vi "Pre Parse Rules.vi"(8 "Error in":errorcluster, 10 "Rules String":string) -> (0 "Error out":errorcluster, 2 "Processed Rules":T1[](array[typedef]))   [LabVIEW 2019, in "LSS.lvlib"]
doc: "Takes the Rules String and splits it into a list of properties that can be used by the property control engine.\n\n<b>Inputs:</b>\n<b>Rules String</b> - Properly formatted string that will control the front panel by applying LSS.\n<b>Error In</b> - Standard Error In terminal.\n\n<b>Outputs:</b>\n<b>Processed Rules</b> - Cluster of criteria and effects that are defined by the Rules String.\n<b>Error Out</b> - Standard Error out terminal."
uses:
  LSS.lvlib
  Controls/Rule.ctl
  Controls/Criteria.ctl
  Controls/Comparison Types.ctl
  Controls/Effects.ctl
panel:
  out "Troubleshooting output only":string[][](array[string])
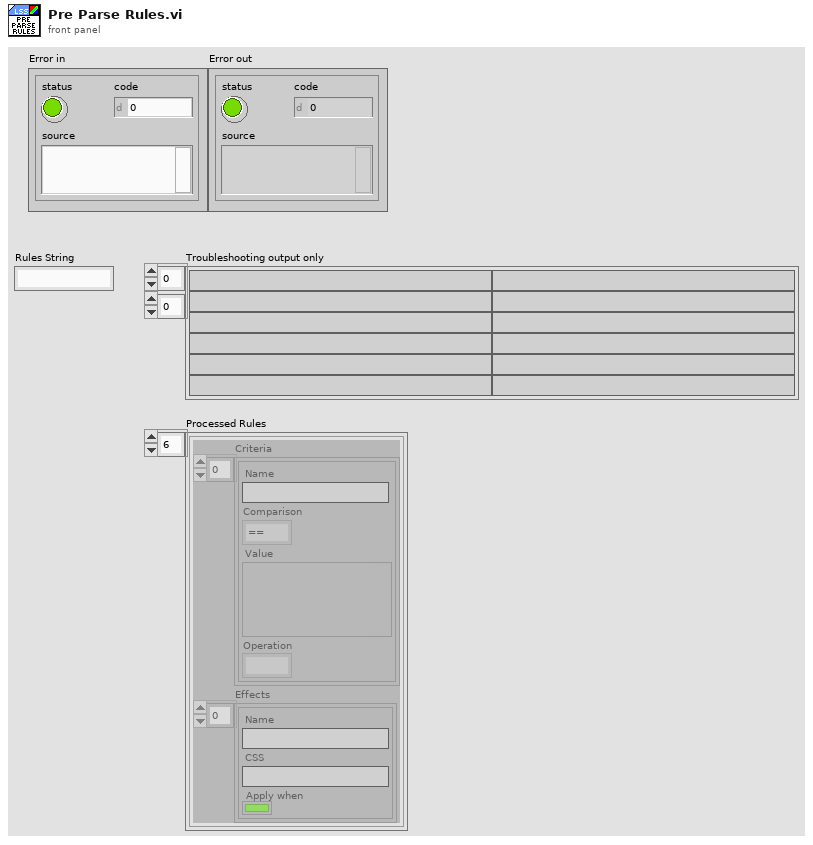
[diagram p1: front panel]
types:
  T1 = typedef "LSS.lvlib/Rule.ctl" = cluster{"Criteria":T2[], "Effects":T4[]}
  T2 = typedef "LSS.lvlib/Criteria.ctl" = cluster{"Name":string, "Comparison":T3, "Value":variant, "Operation":enum16{"Stack", "&&", "||"}}
  T3 = typedef "LSS.lvlib/Comparison Types.ctl" = enum16{"==", "!=", "<", ">", "<=", ">="}
  T4 = typedef "LSS.lvlib/Effects.ctl" = cluster{"Name":string, "CSS":string, "Apply when":bool}
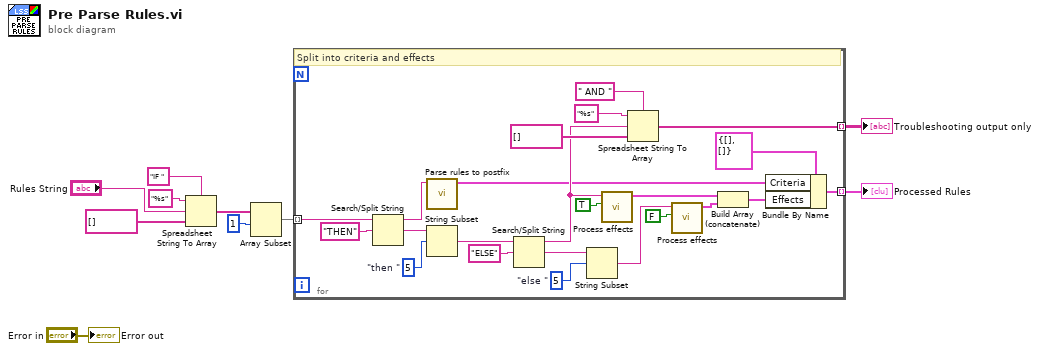
[diagram p0: block diagram]
diagram:
  n1 = Spreadsheet String To Array(delimiter (Tab)="IF ", format string="%s", spreadsheet string="Rules String", array type (2D Dbl)=string[] []) -> (array=w8:string[])
  n2 = Array Subset(array=w8, index=1) -> (w9:string[])  [unwired: 1 in]
  n3 = for {
    tunnel: w9 -> [w32] mode=indexing
    tunnel: [w28] -> w3 mode=indexing
    tunnel: [w20] -> w2 mode=indexing
    w26 = 5  # "else "
    w31 = 5  # "then "
    # "Split into criteria and effects"
    n4 = Search/Split String(string=w32, search string/char (-)="THEN") -> (substring before match=w12:string, match + rest of string=w30:string)  [unwired: 1 in, 1 out]
    n5 = call "Parse rules to postfix.vi"("String"=w12) -> ("Array"=w11:T2[])  [unwired: 10 in]
    n6 = String Subset(string=w30, offset (0)=w31) -> (substring=w25:string)  [unwired: 1 in]
    n7 = Search/Split String(string=w25, search string/char (-)="ELSE") -> (substring before match=w15:string, match + rest of string=w22:string)  [unwired: 1 in, 1 out]
    n8 = String Subset(string=w22, offset (0)=w26) -> (substring=w17:string)  [unwired: 1 in]
    n9 = call "Process effects.vi"("Apply when"=TRUE, "Effect string"=w15) -> ("Effect"=w16:T4[])  [unwired: 9 in]
    n10 = Spreadsheet String To Array(delimiter (Tab)=" AND ", format string="%s", spreadsheet string=w15, array type (2D Dbl)=string[] []) -> (array=w20:string[])
    n11 = call "Process effects.vi"("Apply when"=FALSE, "Effect string"=w17) -> ("Effect"=w23:T4[])  [unwired: 9 in]
    n12 = Build Array (concatenate)(w16, w23) -> (w24:T4[])
    n13 = Bundle By Name(cluster=T1 {"Criteria"=[], "Effects"=[]} ("Cluster"), "Criteria"=w11, "Effects"=w24) -> (w28:T1)
  }
  "Processed Rules" <- w3
  "Troubleshooting output only" <- w2
  "Error out" <- "Error in"
